vi "IsCallCancelled.vi"(8 "error in (no error)":errorcluster, 11 "gRPCid in":T1) -> (0 "error out":errorcluster, 2 "IsCancelled":bool, 3 "gRPCid":T1)   [LabVIEW 2019, in "gprc-support.lvlib"]
uses:
  gprc-support.lvlib
  grpcId.ctl
  build/Debug/labview_grpc_server.dll
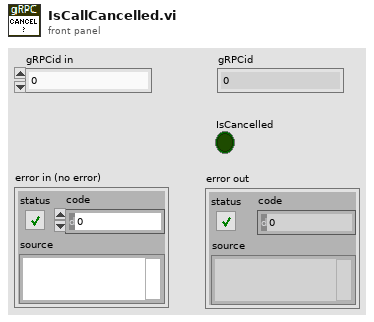
[diagram p1: front panel]
types:
  T1 = typedef "gprc-support.lvlib/grpcId.ctl" = u64
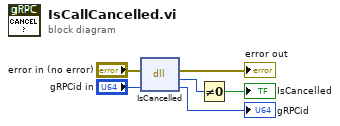
[diagram p0: block diagram]
diagram:
  n1 = dll-call lib="C:/dev/labview-grpc-server/build/Debug/labview_grpc_server.dll" fn="IsCancelled"(error in="error in (no error)", "id"="gRPCid in") -> (error out=→"error out":errorcluster, "return type"=w4:i32, "id"=→"gRPCid":T1)  [unwired: 2 in, 1 out]
  n2 = Not Equal To 0?(x=w4) -> (x != 0?=→"IsCancelled":bool)
